vi "niRFUtil WFM Remove Phase Offset.vi"(0 "Signal In":T1 {"y" format="%.2f"; "dx" format="%^.2e"; "x0" format="%^.2e"}, 5 "Reference Signal In":T1 {"y" format="%.2f"; "dx" format="%^.2e"; "x0" format="%^.2e"}) -> (4 "Signal Out":T1 {"y" format="%.2f"; "dx" format="%^.2e"; "x0" format="%^.2e"}, 6 "Reference Signal Out":T1 {"y" format="%.2f"; "dx" format="%^.2e"; "x0" format="%^.2e"}, 13 "Phase Offset, deg":sgl format="%.2f")   [LabVIEW 2015, in "niRFUtil.lvlib"]
doc: "(c) Copyright 2006, National Instruments, Inc. This VI may not be duplicated, sold, or distributed without written consent from National Instruments."
uses:
  niRFUtil.lvlib
  Includes/niRFUtil INC Complex Waveform.ctl
  Includes/niRFUtil INC Complex Array.ctl
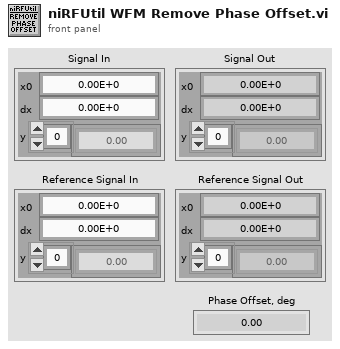
[diagram p1: front panel]
types:
  T1 = typedef "niRFUtil.lvlib/niRFUtil INC Complex Waveform.ctl" = cluster{"x0":dbl, "dx":dbl, "y":T2}
  T2 = typedef "niRFUtil.lvlib/niRFUtil INC Complex Array.ctl" = csg[]
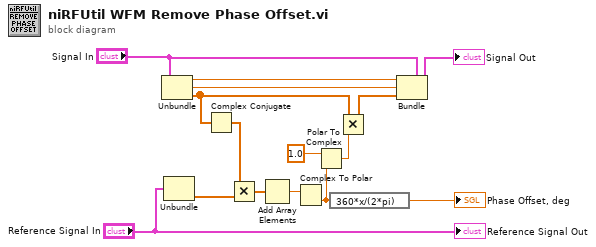
[diagram p0: block diagram]
diagram:
  n1 = Unbundle("Signal In") -> ("x0"=w13:dbl, "dx"=w12:dbl, "y"=w11:T2)
  n2 = Unbundle("Reference Signal In") -> ("y"=w10:T2)  [unwired: 2 out]
  n3 = Complex Conjugate(1:w11) -> (0:w15:T2)
  n4 = Multiply(x=w15, y=w10) -> (x*y=w5:T2)
  n5 = Add Array Elements(numeric array=w5) -> (sum=w1:csg)
  n6 = Complex To Polar(r * e^(i*theta)=w1) -> (theta=w4:sgl)  [unwired: 1 out]
  n7 = Polar To Complex(1:w4, 2:sgl 1.0 ("r")) -> (0:w2:csg)
  n8 = expression code="360*x/(2*pi)"(w4) -> (→"Phase Offset, deg":sgl)
  n9 = Multiply(x=w11, y=w2) -> (x*y=w14:T2)
  n10 = Bundle(cluster="Signal In", "x0"=w13, "dx"=w12, "y"=w14) -> (→"Signal Out":T1)
  "Reference Signal Out" <- "Reference Signal In"
